vi "Simple Obstacle Avoidance.vi"(8 "dt":dbl=100.0, 10 "Lidar Magnitudes":dbl[](array[numeric])=[350.0, 350.0, 350.0, 350.0, 355.0, 355.0, 354.0, 354.0, 353.0, 352.0, 350.0, 350.0, 350.0, 346.0, 346.0, 346.0, 346.0, 350.0, 354.0, 350.0, 350.0, 345.0, 345.0, 345.0, 345.0, 347.0, 347.0, 352.0, 352.0, 349.0, 349.0, 349.0, 347.0, 349.0, 350.0, 347.0, 347.0, 342.0, 340.0, 340.0, 340.0, 342.0, 340.0, 344.0, 341.0, 341.0, 341.0, 341.0, 338.0, 338.0, 338.0, 338.0, 339.0, 339.0, 337.0, 339.0, 337.0, 337.0, 337.0, 343.0, 337.0, 336.0, 343.0, 336.0, 336.0, 339.0, 342.0, 340.0, 340.0, 339.0, 340.0, 339.0, 339.0, 339.0, 342.0, 339.0, 342.0, 342.0, 342.0, 340.0, 348.0, 340.0, 340.0, 340.0, 340.0, 340.0, 340.0, 340.0, 340.0, 338.0, 337.0, 338.0, 339.0, 338.0, 339.0, 341.0, 346.0, 341.0, 345.0, 345.0, 343.0, 340.0, 337.0, 337.0, 340.0, 340.0, 341.0, 347.0, 348.0, 349.0, 349.0, 349.0, 349.0, 349.0, 350.0, 342.0, 349.0, 349.0, 352.0, 349.0, 349.0, 353.0, 350.0, 350.0, 353.0, 353.0, 353.0, 353.0, 353.0, 355.0, 355.0, 355.0, 355.0, 357.0, 357.0, 357.0, 360.0, 360.0, 357.0, 360.0, 360.0, 363.0, 363.0, 363.0, 363.0, 363.0, 365.0, 372.0, 372.0, 372.0, 379.0, 379.0, 385.0, 379.0, 378.0, 378.0, 378.0, 378.0, 384.0, 393.0, 393.0, 394.0, 395.0, 398.0, 402.0, 402.0, 402.0, 402.0, 399.0, 398.0, 398.0, 398.0, 402.0, 409.0, 410.0, 412.0, 412.0, 415.0, 416.0, 416.0, 416.0, 416.0, 420.0, 420.0, 421.0, 428.0, 428.0, 431.0, 435.0, 443.0, 444.0, 443.0, 444.0, 445.0, 446.0, 446.0, 449.0, 456.0, 457.0, 462.0, 466.0, 466.0, 468.0, 475.0, 476.0, 476.0, 482.0, 495.0, 495.0, 495.0, 495.0, 496.0, 497.0, 502.0, 519.0, 522.0, 523.0, 529.0, 529.0, 529.0, 529.0, 535.0, 531.0, 535.0, 551.0, 551.0, 556.0, 559.0, 568.0, 576.0, 582.0, 582.0, 582.0, 582.0, 582.0, 589.0, 601.0, 602.0, 606.0, 614.0, 616.0, 622.0, 622.0, 633.0, 633.0, 651.0, 651.0, 657.0, 661.0, 670.0, 678.0, 684.0, 706.0, 718.0, 725.0, 726.0, 737.0, 761.0, 768.0, 768.0, 793.0, 802.0, 811.0, 828.0, 840.0, 863.0, 873.0, 881.0, 893.0, 914.0, 933.0, 950.0, 971.0, 999.0, 1011.0, 1047.0, 1070.0, 1094.0, 1120.0, 1148.0, 1169.0, 1212.0, 1245.0, 1276.0, 1315.0, 1340.0, 1387.0, 1427.0, 1469.0, 1502.0, 1558.0, 1594.0, 1659.0, 1162.0, 1162.0, 1162.0, 1201.0, 2381.0, 2378.0, 2378.0, 2373.0, 2371.0, 2371.0, 2365.0, 2356.0, 2354.0, 2349.0, 2343.0, 2341.0, 2338.0, 2341.0, 2335.0, 2335.0, 2335.0, 2335.0, 2328.0, 2325.0, 2322.0, 2319.0, 2317.0, 2314.0, 2310.0, 2310.0, 2314.0, 2316.0, 2317.0, 2317.0, 2316.0, 2316.0, 2311.0, 2311.0, 2311.0, 2312.0, 2312.0, 2322.0, 697.0, 673.0, 670.0, 670.0, 670.0, 653.0, 648.0, 653.0, 671.0, 4390.0, 4416.0, 4416.0, 4416.0, 4416.0, 4430.0, 4458.0, 4458.0, 4458.0, 4824.0, 4824.0, 4812.0, 4824.0, 4832.0, 4838.0, 4849.0, 4853.0, 4864.0, 4877.0, 4920.0, 4921.0, 4933.0, 4944.0, 4955.0, 4959.0, 4983.0, 5005.0, 5012.0, 5034.0, 5037.0, 5070.0, 5077.0, 5086.0, 5077.0, 5077.0, 5084.0, 5084.0, 5084.0, 5088.0, 5121.0, 5146.0, 5157.0, 5181.0, 5187.0, 5196.0, 5207.0, 5274.0, 5289.0, 5329.0, 5341.0, 5372.0, 5401.0, 5421.0, 5422.0, 5473.0, 5474.0, 5498.0, 5466.0, 5422.0, 5407.0, 5402.0, 5349.0, 5309.0, 5282.0, 5236.0, 5191.0, 5184.0, 5184.0, 5184.0, 4553.0, 4057.0, 4030.0, 4017.0, 4014.0, 4004.0, 3994.0, 3983.0, 3968.0, 3956.0, 3942.0, 3922.0, 3921.0, 3893.0, 3879.0, 3876.0, 3876.0, 3876.0, 3891.0, 3904.0, 3923.0, 3923.0, 3923.0, 3920.0, 3881.0, 3881.0, 671.0, 668.0, 671.0, 677.0, 671.0, 668.0, 651.0, 649.0, 647.0, 647.0, 647.0, 640.0, 628.0, 626.0, 624.0, 626.0, 624.0, 624.0, 627.0, 627.0, 621.0, 621.0, 621.0, 621.0, 630.0, 633.0, 642.0, 645.0, 645.0, 645.0, 642.0, 636.0, 631.0, 636.0, 636.0, 637.0, 637.0, 637.0, 637.0, 637.0, 637.0, 634.0, 639.0, 642.0, 644.0, 644.0, 654.0, 753.0, 863.0, 871.0, 871.0, 871.0, 859.0, 859.0, 849.0, 846.0, 837.0, 836.0, 836.0, 837.0, 862.0, 864.0, 3645.0, 3645.0, 3645.0, 3615.0, 3608.0, 3600.0, 3600.0, 3615.0, 3571.0, 3680.0, 3680.0, 1162.0, 1124.0, 1124.0, 1124.0, 1124.0, 1124.0, 1115.0, 1108.0, 1102.0, 1096.0, 1096.0, 1092.0, 1088.0, 1081.0, 1067.0, 1067.0, 1049.0, 1049.0, 1049.0, 1049.0, 1049.0, 1049.0, 1035.0, 1007.0, 993.0, 987.0, 987.0, 987.0, 1004.0, 1005.0, 1006.0, 1006.0, 1006.0, 1012.0, 1006.0, 1006.0, 1014.0, 1014.0, 1052.0, 1052.0, 1052.0, 1047.0, 1046.0, 1045.0, 1045.0, 1042.0, 1042.0, 1042.0, 1034.0, 1034.0, 1047.0, 1048.0, 1048.0, 1062.0, 1092.0, 1100.0, 1106.0, 1106.0, 1106.0, 1107.0, 1115.0, 1144.0, 1182.0, 1189.0, 1218.0, 1239.0, 1262.0, 1273.0, 159.8691262202886], 11 "Lidar Angles":dbl[](array[numeric])=[1.9164533309984608, 1.9103174078469183, 1.9041814846953757, 1.8980455615438332, 1.8919096383922906, 1.885773715240748, 1.8796377920892056, 1.873501868937663, 1.8673659457861205, 1.861230022634578, 1.8550940994830352, 1.8489581763314926, 1.84282225317995, 1.8366863300284075, 1.830550406876865, 1.8244144837253224, 1.81827856057378, 1.8121426374222374, 1.8060067142706948, 1.7998707911191523, 1.7937348679676097, 1.787598944816067, 1.7814630216645244, 1.7753270985129819, 1.7691911753614393, 1.7630552522098968, 1.7569193290583542, 1.7507834059068117, 1.7446474827552692, 1.7385115596037266, 1.732375636452184, 1.7262397133006415, 1.7201037901490988, 1.7139678669975562, 1.7078319438460137, 1.7016960206944711, 1.6955600975429286, 1.689424174391386, 1.6832882512398435, 1.677152328088301, 1.6710164049367584, 1.6648804817852159, 1.658744558633673, 1.6526086354821306, 1.646472712330588, 1.6403367891790455, 1.634200866027503, 1.6280649428759604, 1.6219290197244178, 1.6157930965728753, 1.6096571734213327, 1.6035212502697902, 1.5973853271182477, 1.591249403966705, 1.5851134808151623, 1.5789775576636198, 1.5728416345120773, 1.566705711360535, 1.5605697882089924, 1.5544338650574498, 1.5482979419059073, 1.5421620187543645, 1.536026095602822, 1.5298901724512795, 1.523754249299737, 1.5176183261481944, 1.5114824029966518, 1.5053464798451093, 1.4992105566935667, 1.4930746335420242, 1.4869387103904816, 1.480802787238939, 1.4746668640873963, 1.4685309409358538, 1.4623950177843112, 1.4562590946327687, 1.4501231714812262, 1.4439872483296836, 1.437851325178141, 1.4317154020265985, 1.425579478875056, 1.4194435557235134, 1.413307632571971, 1.4071717094204281, 1.4010357862688856, 1.394899863117343, 1.3887639399658005, 1.382628016814258, 1.3764920936627154, 1.3703561705111729, 1.3642202473596303, 1.3580843242080878, 1.3519484010565452, 1.3458124779050025, 1.33967655475346, 1.3335406316019174, 1.3274047084503748, 1.3212687852988323, 1.3151328621472897, 1.3089969389957472, 1.3028610158442047, 1.2967250926926621, 1.2905891695411196, 1.284453246389577, 1.2783173232380343, 1.2721814000864917, 1.2660454769349492, 1.2599095537834066, 1.253773630631864, 1.2476377074803215, 1.241501784328779, 1.2353658611772365, 1.229229938025694, 1.2230940148741514, 1.2169580917226088, 1.210822168571066, 1.2046862454195235, 1.198550322267981, 1.1924143991164384, 1.1862784759648959, 1.1801425528133533, 1.1740066296618108, 1.1678707065102683, 1.1617347833587257, 1.1555988602071832, 1.1494629370556404, 1.1433270139040979, 1.1371910907525553, 1.1310551676010128, 1.1249192444494702, 1.1187833212979277, 1.1126473981463851, 1.1065114749948426, 1.1003755518433, 1.0942396286917575, 1.088103705540215, 1.0819677823886722, 1.0758318592371297, 1.069695936085587, 1.0635600129340446, 1.057424089782502, 1.0512881666309595, 1.045152243479417, 1.0390163203278744, 1.0328803971763318, 1.0267444740247893, 1.0206085508732468, 1.014472627721704, 1.0083367045701614, 1.002200781418619, 0.9960648582670764, 0.9899289351155338, 0.9837930119639913, 0.9776570888124487, 0.9715211656609062, 0.9653852425093635, 0.959249319357821, 0.9531133962062784, 0.9469774730547359, 0.9408415499031934, 0.9347056267516507, 0.9285697036001082, 0.9224337804485656, 0.9162978572970231, 0.9101619341454805, 0.9040260109939379, 0.8978900878423953, 0.8917541646908528, 0.8856182415393102, 0.8794823183877677, 0.8733463952362251, 0.8672104720846825, 0.86107454893314, 0.8549386257815974, 0.8488027026300549, 0.8426667794785123, 0.8365308563269697, 0.8303949331754271, 0.8242590100238846, 0.818123086872342, 0.8119871637207995, 0.8058512405692568, 0.7997153174177143, 0.7935793942661717, 0.7874434711146292, 0.7813075479630865, 0.775171624811544, 0.7690357016600015, 0.7628997785084588, 0.7567638553569163, 0.7506279322053737, 0.7444920090538312, 0.7383560859022886, 0.732220162750746, 0.7260842395992034, 0.7199483164476609, 0.7138123932961183, 0.7076764701445758, 0.7015405469930333, 0.6954046238414906, 0.689268700689948, 0.6831327775384055, 0.676996854386863, 0.6708609312353204, 0.6647250080837778, 0.6585890849322352, 0.6524531617806927, 0.6463172386291501, 0.6401813154776076, 0.6340453923260649, 0.6279094691745224, 0.6217735460229799, 0.6156376228714373, 0.6095016997198948, 0.6033657765683522, 0.5972298534168096, 0.591093930265267, 0.5849580071137245, 0.5788220839621819, 0.5726861608106394, 0.5665502376590967, 0.5604143145075542, 0.5542783913560116, 0.5481424682044691, 0.5420065450529266, 0.5358706219013839, 0.5297346987498414, 0.5235987755982988, 0.5174628524467563, 0.5113269292952137, 0.5051910061436712, 0.4990550829921286, 0.492919159840586, 0.48678323668904344, 0.4806473135375009, 0.4745113903859583, 0.46837546723441575, 0.46223954408287315, 0.4561036209313306, 0.44996769777978807, 0.44383177462824547, 0.4376958514767029, 0.4315599283251604, 0.4254240051736178, 0.41928808202207524, 0.41315215887053264, 0.4070162357189901, 0.40088031256744755, 0.39474438941590495, 0.38860846626436246, 0.38247254311281986, 0.3763366199612773, 0.3702006968097348, 0.3640647736581922, 0.35792885050664963, 0.35179292735510703, 0.3456570042035645, 0.33952108105202194, 0.33338515790047935, 0.3272492347489368, 0.32111331159739426, 0.31497738844585166, 0.3088414652943091, 0.3027055421427665, 0.29656961899122397, 0.2904336958396814, 0.28429777268813883, 0.2781618495365963, 0.27202592638505374, 0.26589000323351114, 0.2597540800819686, 0.253618156930426, 0.24748223377888345, 0.24134631062734088, 0.23521038747579834, 0.22907446432425577, 0.2229385411727132, 0.21680261802117062, 0.21066669486962808, 0.2045307717180855, 0.19839484856654294, 0.19225892541500036, 0.1861230022634578, 0.17998707911191522, 0.17385115596037265, 0.1677152328088301, 0.16157930965728753, 0.15544338650574496, 0.1493074633542024, 0.14317154020265985, 0.13703561705111728, 0.1308996938995747, 0.12476377074803215, 0.10022007814186189, 0.09408415499031933, 0.08794823183877676, 0.0818123086872342, 0.05726861608106394, 0.05113269292952138, 0.044996769777978805, 0.03886084662643624, 0.032724923474893676, 0.02658900032335111, 0.02045307717180855, 0.014317154020265985, 0.008181230868723419, 0.0020453077171808547, -0.0040906154343617095, -0.010226538585904275, -0.016362461737446838, -0.022498384888989403, -0.02863430804053197, -0.034770231192074535, -0.0409061543436171, -0.047042077495159665, -0.05317800064670222, -0.05931392379824479, -0.06544984694978735, -0.07158577010132992, -0.07772169325287248, -0.08385761640441505, -0.08999353955595761, -0.09612946270750018, -0.10226538585904275, -0.10840130901058531, -0.11453723216212788, -0.12067315531367044, -0.126809078465213, -0.13294500161675557, -0.13908092476829814, -0.1452168479198407, -0.15135277107138326, -0.15748869422292583, -0.1636246173744684, -0.16976054052601097, -0.19430423313218123, -0.20044015628372377, -0.20657607943526632, -0.2127120025868089, -0.21884792573835146, -0.22498384888989403, -0.23111977204143658, -0.23725569519297915, -0.24339161834452172, -0.2495275414960643, -0.25566346464760686, -0.2617993877991494, -0.26793531095069195, -0.27407123410223455, -0.2802071572537771, -0.2863430804053197, -0.3047508498599474, -0.3108867730114899, -0.4274693128907987, -0.43360523604234125, -0.43974115919388385, -0.4458770823454264, -0.45201300549696893, -0.45814892864851153, -0.4642848518000541, -0.4704207749515967, -0.4765566981031392, -0.48269262125468176, -0.48882854440622436, -0.4949644675577669, -0.5011003907093095, -0.507236313860852, -0.5133722370123946, -0.5195081601639372, -0.5256440833154797, -0.5317800064670223, -0.5379159296185648, -0.5440518527701075, -0.55018777592165, -0.5563236990731926, -0.5624596222247351, -0.5685955453762777, -0.5747314685278202, -0.5808673916793629, -0.5870033148309054, -0.5931392379824479, -0.5992751611339905, -0.605411084285533, -0.6115470074370757, -0.6176829305886182, -0.6238188537401608, -0.6299547768917033, -0.6360907000432459, -0.6422266231947885, -0.6483625463463311, -0.6544984694978736, -0.6606343926494161, -0.6667703158009587, -0.6729062389525012, -0.6790421621040439, -0.6851780852555864, -0.691314008407129, -0.6974499315586715, -0.7035858547102141, -0.7097217778617567, -0.7158577010132993, -0.7833528556802675, -0.7894887788318099, -0.7956247019833524, -0.8017606251348951, -0.8078965482864376, -0.8140324714379802, -0.8201683945895227, -0.8263043177410653, -0.8324402408926079, -0.8385761640441505, -0.844712087195693, -0.8508480103472356, -0.8999353955595761, -0.9060713187111187, -0.9122072418626612, -0.9183431650142038, -0.9244790881657463, -0.930615011317289, -0.9367509344688315, -0.942886857620374, -0.9490227807719166, -0.9551587039234591, -0.9612946270750018, -0.9674305502265443, -0.9735664733780869, -0.9797023965296294, -0.985838319681172, -0.9919742428327145, -0.9981101659842572, -1.0042460891357996, -1.0103820122873424, -1.016517935438885, -1.0226538585904275, -1.02878978174197, -1.0349257048935125, -1.041061628045055, -1.0471975511965976, -1.0533334743481402, -1.0594693974996827, -1.0656053206512253, -1.0717412438027678, -1.0778771669543106, -1.0840130901058531, -1.0901490132573957, -1.0962849364089382, -1.1024208595604807, -1.1085567827120233, -1.1146927058635658, -1.1208286290151084, -1.126964552166651, -1.1331004753181935, -1.139236398469736, -1.1453723216212788, -1.1515082447728213, -1.1576441679243639, -1.1637800910759064, -1.169916014227449, -1.1760519373789915, -1.182187860530534, -1.1883237836820766, -1.1944597068336191, -1.2005956299851617, -1.2067315531367044, -1.212867476288247, -1.2190033994397895, -1.225139322591332, -1.2312752457428746, -1.2374111688944172, -1.2435470920459597, -1.2496830151975022, -1.2558189383490448, -1.2619548615005873, -1.2680907846521299, -1.2742267078036726, -1.2803626309552152, -1.2864985541067577, -1.2926344772583003, -1.2987704004098428, -1.3049063235613854, -1.311042246712928, -1.3171781698644704, -1.323314093016013, -1.3294500161675555, -1.335585939319098, -1.3417218624706408, -1.3478577856221834, -1.353993708773726, -1.3601296319252685, -1.366265555076811, -1.3724014782283536, -1.378537401379896, -1.3846733245314387, -1.3908092476829812, -1.3969451708345237, -1.4030810939860665, -1.409217017137609, -1.4153529402891516, -1.4214888634406941, -1.4276247865922367, -1.4337607097437792, -1.4398966328953218, -1.4460325560468643, -1.4521684791984069, -1.4583044023499494, -1.464440325501492, -1.4705762486530347, -1.4767121718045773, -1.4828480949561198, -1.4889840181076623, -1.4951199412592049, -1.5012558644107474, -1.50739178756229, -1.5135277107138325, -1.519663633865375, -1.5257995570169176, -1.5319354801684602, -1.538071403320003, -1.5442073264715455, -1.550343249623088, -1.5564791727746305, -1.562615095926173, -1.5687510190777156, -1.5748869422292584, -1.581022865380801, -1.5871587885323435, -1.593294711683886, -1.5994306348354286, -1.6055665579869711, -1.6117024811385137, -1.6178384042900564, -1.623974327441599, -1.6301102505931415, -1.636246173744684, -1.6423820968962266, -1.6485180200477692, -1.6546539431993117, -1.6607898663508542, -1.6669257895023968, -1.6730617126539393, -1.679197635805482, -1.6853335589570246, -1.6914694821085672, -1.6976054052601097, -1.7037413284116523, -1.7098772515631948, -1.7160131747147374, -1.72214909786628, -1.7282850210178224, -1.734420944169365, -1.7405568673209075, -1.7466927904724503, -1.7528287136239928, -1.7589646367755354, -1.765100559927078, -1.7712364830786205, -1.777372406230163, -1.7835083293817056, -1.789644252533248, -1.7957801756847906, -1.8019160988363332, -1.8080520219878757, -1.8141879451394185, -1.820323868290961, -1.8264597914425036, -1.8325957145940461, -1.8387316377455887, -1.8448675608971312, -1.8510034840486738, -1.8571394072002163, -1.8632753303517589, -1.8694112535033014, -1.8755471766548442, -1.8816830998063867, -1.8878190229579292, -1.8939549461094718, -1.9000908692610143, -1.9062267924125569, -1.9123627155640994, -1.918498638715642]) -> (3 "New wall following distance":dbl=230.0)   [LabVIEW 2017]
uses:
  Globals/Pose.vi
panel:
  in  "Wall Left?":bool=TRUE
  out "Maximum distance to look 2":dbl=650.0
  out "XY Graph 2":cluster{i32[], dbl[]}(graph)={[0, 1, 2, 3, 4, 5, 6, 7, 8, 9, 10, 11, 12, 13, 14, 15, 16, 17, 18, 19, 20, 21, 22, 23, 24, 25, 26, 27, 28, 29, 30, 31, 32, 33, 34, 35, 36, 37, 38, 39], [4.773148796175519e-05, 8.908076811731114e-05, 0.0004775492338182641, 0.00022136510783621333, 0.0010874017334057129, 0.0008005965494133349, 0.0003859678677766709, 0.23097157477187125, 1.2233006080312974, 2.2233006080312974, 3.2233006080312974, 4.223300608031297, 5.223300608031297, 6.223300608031297, 7.223300608031297, 8.223300608031298, 9.223300608031298, 10.223300608031298, 11.223300608031298, 12.223300608031298, 13.223300608031298, 14.223300608031298, 15.230971574771871, 16.23097157477187, 16.202283468588057, 15.202283468588057, 14.202283468588057, 13.202283468588057, 12.202283468588057, 11.202283468588057, 10.202283468588057, 9.202283468588057, 8.202283468588057, 7.202283468588057, 6.202283468588057, 5.202283468588057, 4.202283468588057, 3.202283468588057, 2.202283468588057, 1.2022834685880568]}
  out "distances of obstacles":cluster{i32[], dbl[]}(graph)={[0, 1, 2, 3, 4, 5, 6, 7, 8, 9, 10, 11, 12, 13, 14, 15, 16, 17, 18, 19, 20, 21, 22, 23, 24, 25, 26, 27, 28, 29, 30, 31, 32, 33, 34, 35, 36, 37, 38, 39], [4.773148796175519e-05, 8.908076811731114e-05, 0.0004775492338182641, 0.00022136510783621333, 0.0010874017334057129, 0.0008005965494133349, 0.0003859678677766709, 0.23097157477187125, 1.2233006080312974, 2.2233006080312974, 3.2233006080312974, 4.223300608031297, 5.223300608031297, 6.223300608031297, 7.223300608031297, 8.223300608031298, 9.223300608031298, 10.223300608031298, 11.223300608031298, 12.223300608031298, 13.223300608031298, 14.223300608031298, 15.230971574771871, 16.23097157477187, 16.202283468588057, 15.202283468588057, 14.202283468588057, 13.202283468588057, 12.202283468588057, 11.202283468588057, 10.202283468588057, 9.202283468588057, 8.202283468588057, 7.202283468588057, 6.202283468588057, 5.202283468588057, 4.202283468588057, 3.202283468588057, 2.202283468588057, 1.2022834685880568]}
  in  "Column Blocked time":dbl=4000.0 format="%#_13g"
  in  "Wall margin (cm)":dbl=10.0
  out "LIDAR Data":cluster{dbl[], dbl[]}(graph)
  in  "Maximum distance to look":dbl=750.0
  in  "Collision radius (mm)":dbl=100.0
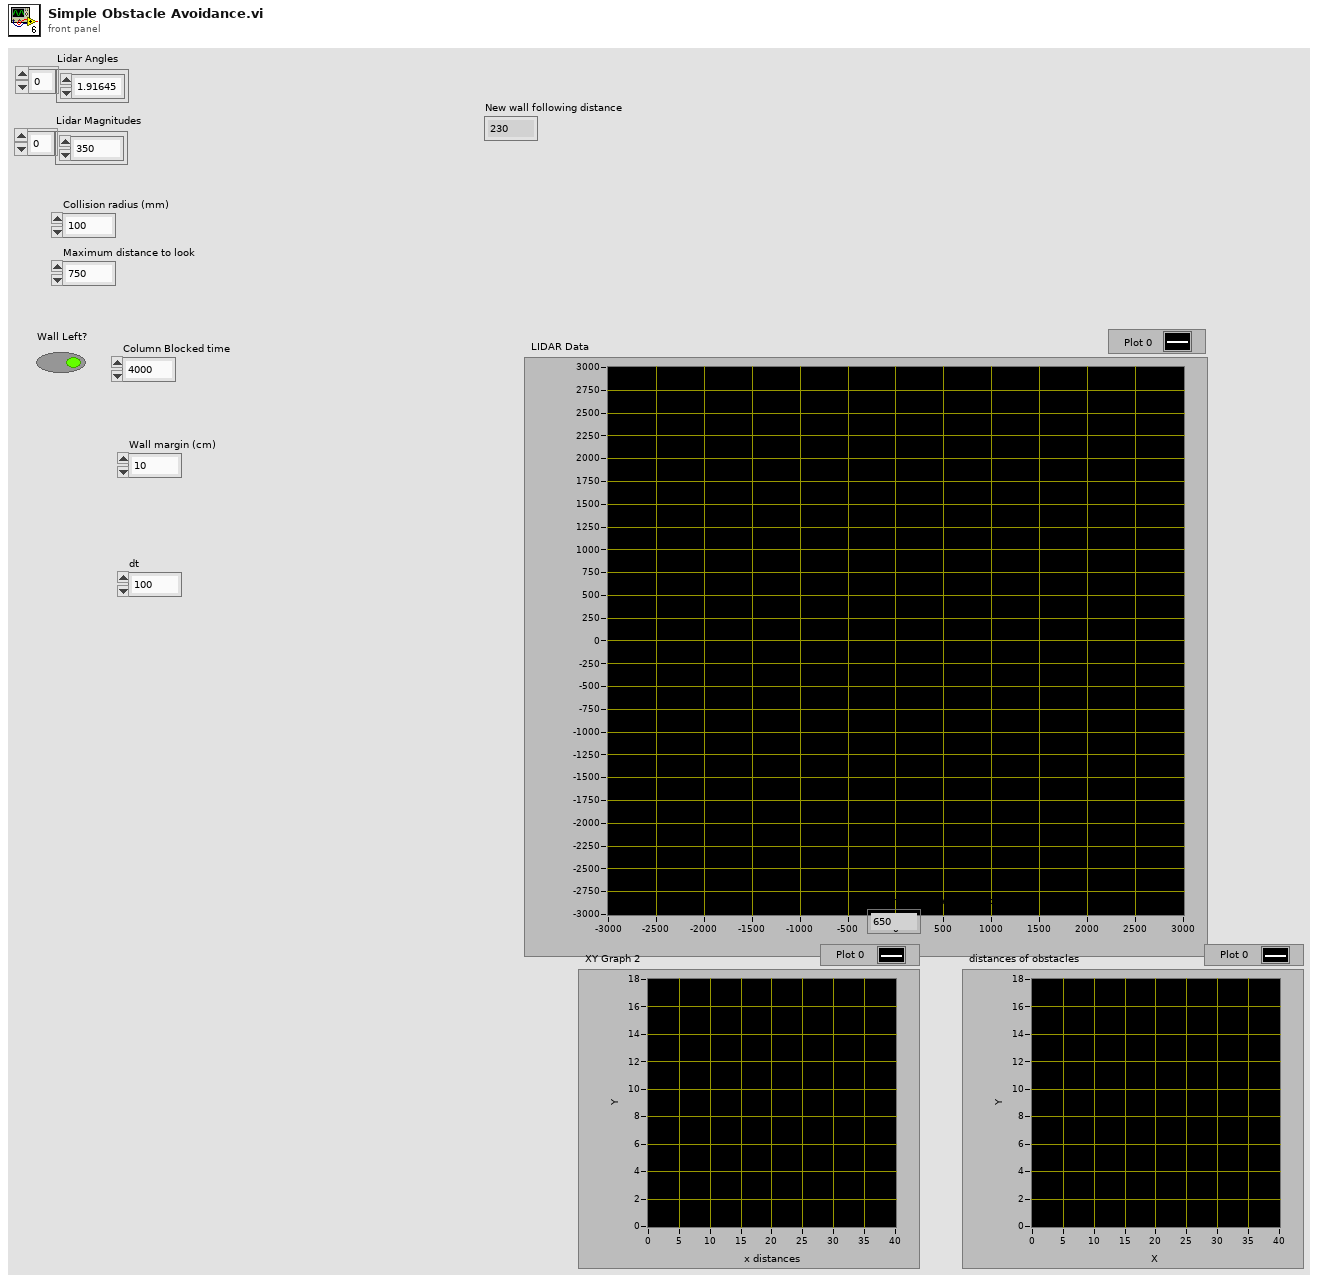
[diagram p1: front panel]
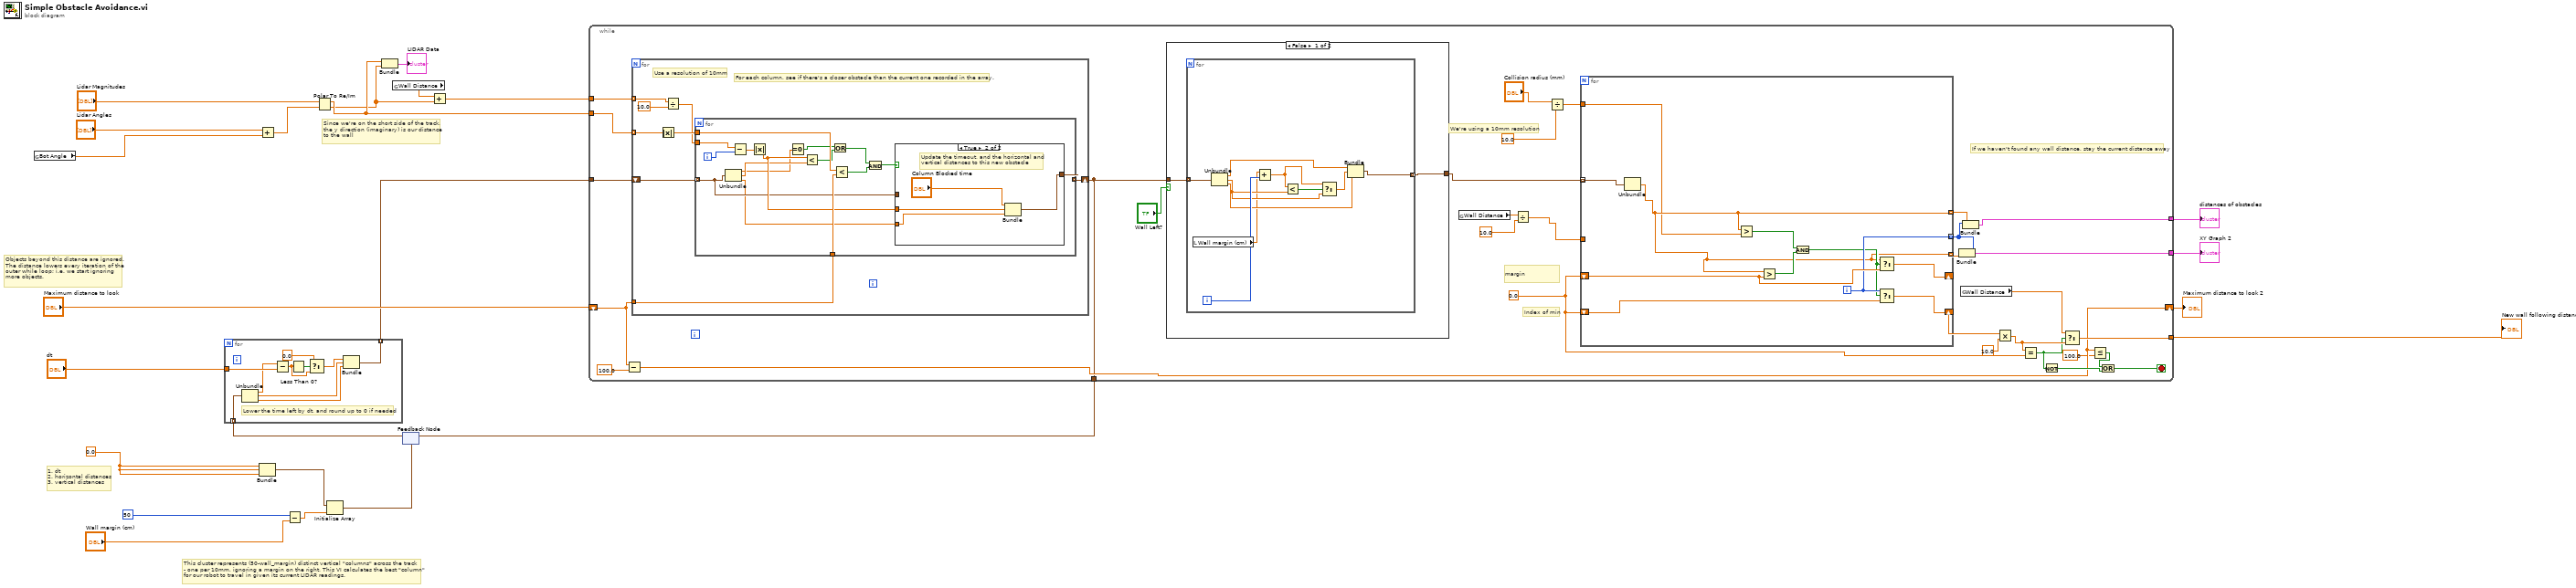
[diagram p0: block diagram]
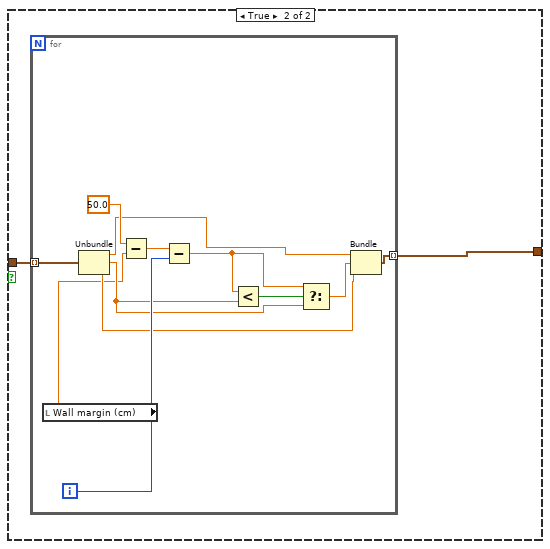
[diagram p2: hidden frame]
diagram:
  w5 = 0.0
  # "Objects beyond this distance are ignored.\nThe distance lowers every iteration of the\nouter while loop; i.e. we start ignoring \nmore objects."
  # "This cluster represents (50-wall_margin) distinct vertical \"columns\" across the track\n- one per 10mm, ignoring a margin on the right. This VI calculates the best \"column\"\nfor our robot to travel in given its current LIDAR readings."
  # "1. dt\n2. horizontal distances\n3. vertical distances"
  # "Since we're on the short side of the track,\nthe y direction (imaginary) is our distance\nto the wall"
  n1 = global read "Pose.vi" "Bot Angle"() -> (w17:dbl)
  n2 = Bundle(w5, w5, w5) -> (w9:cluster{dbl, dbl, dbl})  [unwired: 1 in]
  n3 = Add(x="Lidar Angles", y=w17) -> (x+y=w16:dbl[])
  n4 = Subtract(x=50 ("dimension size"), y="Wall margin (cm)") -> (x-y=w10:dbl)
  n5 = Polar To Re/Im(2:w16, 3:"Lidar Magnitudes") -> (0:w14:dbl[], 1:w15:dbl[])
  n6 = Initialize Array(w9, w10) -> (w8:cluster{dbl, dbl, dbl}[])
  n7 = Bundle(w15, w14) -> (→"LIDAR Data":cluster{dbl[], dbl[]})  [unwired: 1 in]
  n8 = global read "Pose.vi" "Wall Distance"() -> (w23:dbl)
  n9 = feedback #1(w8) -> (w7:cluster{dbl, dbl, dbl}[])
  n10 = for {
    tunnel: "dt" -> [w34]
    tunnel: w7 -> [w30] mode=indexing
    tunnel: [w26] -> w6 mode=indexing
    # "Lower the time left by dt, and round up to 0 if needed"
    n11 = Unbundle(w30) -> (w29:dbl, w27:dbl, w25:dbl)
    n12 = Subtract(x=w29, y=w34) -> (x-y=w31:dbl)
    n13 = Less Than 0?(x=w31) -> (x < 0?=w33:bool)
    n14 = Select(t=0.0, s=w33, f=w31) -> (s? t:f=w28:dbl)
    n15 = Bundle("t"=w28, w27, w25) -> (w26:cluster{"t":dbl, dbl, dbl})  [unwired: 1 in]
  }
  n16 = Add(x=w23, y=w14) -> (x+y=w22:dbl[])
  n17 = while {
    tunnel: w22 -> [w65]
    tunnel: [w47] -> w19
    tunnel: w15 -> [w62]
    tunnel: w6 -> [w59]
    tunnel: [w37] -> w4
    shift-right: [w43] -> w3
    shift-left: "Maximum distance to look" -> [w45]
    tunnel: [w39] -> w2
    tunnel: [w38] -> w1
    stop <- w40 stop-if-true
    w64 = 0.0
    # "Index of min"
    # "margin"
    # "We're using a 10mm resolution"
    # "If we haven't found any wall distance, stay the current distance away"
    n18 = Subtract(x=w45, y=100.0) -> (x-y=w43:dbl)
    n19 = for {
      tunnel: w65 -> [w110] mode=indexing
      shift-right: [w104] -> w37
      shift-left: w59 -> [w108]
      tunnel: w45 -> [w107]
      tunnel: w62 -> [w106] mode=indexing
      # "For each column, see if there's a closer obstacle than the current one recorded in the array."
      # "Use a resolution of 10mm"
      n20 = Absolute Value(x=w106) -> (abs(x)=w105:dbl)
      n21 = Divide(x=w110, y=10.0) -> (x/y=w103:dbl)
      n22 = for {
        tunnel: w103 -> [w126]
        tunnel: w108 -> [w118] mode=indexing
        tunnel: w107 -> [w124]
        tunnel: w105 -> [w123]
        tunnel: [w116] -> w104 mode=indexing
        i -> [w125]
        n23 = Unbundle(w118) -> ("t"=w112:dbl, w117:dbl, w111:dbl)
        n24 = Subtract(x=w126, y=w125) -> (x-y=w119:dbl)
        n25 = Absolute Value(x=w119) -> (abs(x)=w120:dbl)
        n26 = Equal To 0?(x=w112) -> (x = 0?=w113:bool)
        n27 = Less?(x=w120, y=w117) -> (x < y?=w114:bool)
        n28 = Or(x=w113, y=w114) -> (x .or. y?=w115:bool)
        n29 = Less?(x=w123, y=w124) -> (x < y?=w122:bool)
        n30 = And(x=w115, y=w122) -> (x .and. y?=w121:bool)
        n31 = case shown="True" w121 {
          tunnel: w120 -> [_ w129]
          tunnel: w118 -> [w127 _]
          tunnel: [w127 w130] -> w116
          tunnel: w111 -> [_ w128]
          frame False {
          }
          frame True {
            # "Update the timeout, and the horizontal and\nvertical distances to this new obstacle"
            n32 = Bundle("Column Blocked time"="Column Blocked time", w129, w128) -> (w130:cluster{"Column Blocked time":dbl, dbl, dbl})  [unwired: 1 in]
          }
        }
      }
    }
    n33 = case shown="False" "Wall Left?" {
      tunnel: w37 -> [w67 w79]
      tunnel: [w66 w78] -> w35
      frame False {
        n34 = for {
          tunnel: w67 -> [w77] mode=indexing
          tunnel: [w69] -> w66 mode=indexing
          i -> [w76]
          n35 = local read "Wall margin (cm)"() -> (w68:dbl)
          n36 = Unbundle(w77) -> ("t"=w72:dbl, w71:dbl, w70:dbl)
          n37 = Add(x=w68, y=w76) -> (x+y=w73:dbl)
          n38 = Less?(x=w73, y=w71) -> (x < y?=w75:bool)
          n39 = Select(t=w73, s=w75, f=w71) -> (s? t:f=w74:dbl)
          n40 = Bundle("t"=w72, w74, w70) -> (w69:cluster{"t":dbl, dbl, dbl})  [unwired: 1 in]
        }
      }
      frame True {
        n41 = for {
          tunnel: w79 -> [w91] mode=indexing
          tunnel: [w81] -> w78 mode=indexing
          i -> [w88]
          n42 = local read "Wall margin (cm)"() -> (w80:dbl)
          n43 = Unbundle(w91) -> ("t"=w86:dbl, w87:dbl, w82:dbl)
          n44 = Subtract(x=50.0 ("y"), y=w80) -> (x-y=w89:dbl)
          n45 = Subtract(x=w89, y=w88) -> (x-y=w84:dbl)
          n46 = Less?(x=w84, y=w87) -> (x < y?=w85:bool)
          n47 = Select(t=w84, s=w85, f=w87) -> (s? t:f=w83:dbl)
          n48 = Bundle("t"=w86, w83, w82) -> (w81:cluster{"t":dbl, dbl, dbl})  [unwired: 1 in]
        }
      }
    }
    n49 = global read "Pose.vi" "Wall Distance"() -> (w52:dbl)
    n50 = Divide(x=w52, y=10.0) -> (x/y=w49:dbl)
    n51 = Divide(x="Collision radius (mm)", y=10.0) -> (x/y=w50:dbl)
    n52 = for {
      tunnel: w35 -> [w102] mode=indexing
      tunnel: w49 -> [_]
      shift-right: [w101] -> _
      shift-left: w64 -> [w99]
      shift-right: [w100] -> w58
      shift-left: w64 -> [w98]
      tunnel: w50 -> [w93]
      tunnel: [w94] -> w57 mode=indexing
      tunnel: [w97] -> w56 mode=indexing
      tunnel: [w94] -> w55 mode=indexing
      i -> [w97]
      n53 = Unbundle(w102) -> (w94:dbl)  [unwired: 2 out]
      n54 = Greater?(x=w94, y=w93) -> (0:w92:bool)
      n55 = Greater?(x=w94, y=w99) -> (0:w95:bool)
      n56 = And(x=w92, y=w95) -> (x .and. y?=w96:bool)
      n57 = Select(t=w94, s=w96, f=w99) -> (s? t:f=w101:dbl)
      n58 = Select(t=w97, s=w96, f=w98) -> (s? t:f=w100:dbl)
    }
    n59 = Bundle(w56, w55) -> (w38:cluster{i32[], dbl[]})  [unwired: 1 in]
    n60 = global read "Pose.vi" "Wall Distance"() -> (w63:dbl)
    n61 = Bundle(w56, w57) -> (w39:cluster{i32[], dbl[]})  [unwired: 1 in]
    n62 = Multiply(x=w58, y=10.0) -> (x*y=w60:dbl)
    n63 = Equal?(x=w60, y=w64) -> (x = y?=w48:bool)
    n64 = Not(x=w48) -> (.not. x?=w44:bool)
    n65 = Select(t=w63, s=w48, f=w60) -> (s? t:f=w47:dbl)
    n66 = Less Or Equal?(x=w43, y=100.0) -> (x <= y?=w41:bool)
    n67 = Or(x=w41, y=w44) -> (x .or. y?=w40:bool)
  }
  "New wall following distance" <- w19
  "Maximum distance to look 2" <- w3
  "distances of obstacles" <- w2
  "XY Graph 2" <- w1
  n68 = feedback-in #1(w4) -> ()
